vi "Status_Ref_API.vi"(0 "DVR In":refnum<data-value>, 11 "Error In":errorcluster) -> (4 "DVR Out":refnum<data-value>, 6 "VI Ref":refnum<vi>, 15 "Error Out":errorcluster)   [LabVIEW 2020, in "Test.lvclass"]
doc: "Status Reference API"
uses:
  Test.lvclass
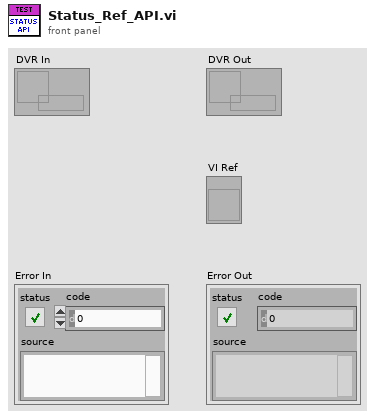
[diagram p1: front panel]
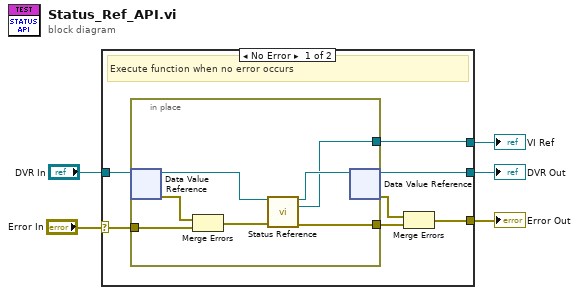
[diagram p0: block diagram]
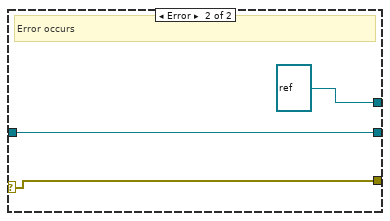
[diagram p2: hidden frame]
diagram:
  n1 = case shown="No Error" "Error In" {
    selector: "Error In" -> [w12 w20]
    tunnel: "DVR In" -> [w11 w21]
    tunnel: [w10 refnum<vi> refnum ("VI ref")] -> w1
    tunnel: [w9 w21] -> w2
    tunnel: [w6 w20] -> w3
    frame No Error {
      # "Execute function when no error occurs"
      n2 = in-place {
        in-place-border: w12 -> [w19]
        in-place-border: [w14] -> w10
        in-place-border: [w13] -> w7
        n3 = in-place-dvr #1(w11) -> (w16:refnum<class "Test.lvclass">, w18:errorcluster)
        n4 = Merge Errors(w18, w19) -> (w17:errorcluster)
        n5 = call-dynamic "Status Reference.vi"("Test in"=w16, "Error in"=w17) -> ("Test out"=w15:refnum<class "Test.lvclass">, "VI ref"=w14:refnum<vi>, "Error out"=w13:errorcluster)  [unwired: 11 in]
        n6 = in-place-dvr #1(w15) -> (w9:refnum<data-value>, w8:errorcluster)
      }
      n7 = Merge Errors(w8, w7) -> (w6:errorcluster)
    }
    frame Error {
      # "Error occurs"
    }
  }
  "Error Out" <- w3
  "DVR Out" <- w2
  "VI Ref" <- w1
